vi "Main.vi"() -> ()   [LabVIEW 2013]
uses:
  <vilib>/Platform/TimedLoop/XDataNode/timing_clust.ctl
  <vilib>/Platform/TimedLoop/XDataNode/nitl_modes.ctl
  <vilib>/Platform/TimedLoop/XDataNode/wakeup.ctl
  <vilib>/DAQmx/read.llb/DAQmx Read (Analog 1D Wfm NChan NSamp).vi
  <vilib>/Analysis/2dsp.llb/Real FFT.vi
  <vilib>/DAQmx/create/channels.llb/DAQmx Create Channel (AI-Voltage-Basic).vi
  <vilib>/DAQmx/configure/timing.llb/DAQmx Timing (Sample Clock).vi
  <vilib>/addons/database/Connection.llb/DB Tools Open Connec (Path).vi
  <vilib>/Waveform/WDTOps.llb/WDT Index Channel DBL.vi
  <vilib>/measure/mamon.llb/Trigger Detection for 1 Channel.vi
  <vilib>/Waveform/WDTOps.llb/WDT Get Waveform Subset DBL.vi
  <vilib>/DAQmx/miscellaneous.llb/DAQmx Fill In Error Info.vi
  <vilib>/platform/TimedLoop/XDataNode/XDataNode.xnode
  <vilib>/addons/database/_DB Variant To Data/Database Variant To Data.xnode
  <vilib>/measure/NI_MAPro.lvlib
  <resource>/objmgr/daqmx.rc
  <vilib>/Analysis/NI_AALPro.lvlib
  <vilib>/addons/database/NI_Database_API.lvlib
  <vilib>/Platform/TimedLoop/XDataNode/XDNodeRunTimeDep.lvlib
panel:
  out "FFT 2":cluster{"t":dbl, dbl, dbl[]}(graph)
  in  "Canal 2":enum32{"DB"}(tab)
  in  "DB Retrieve 2":bool
  in  "Tabla 3":u16(ring) items=["Mediciones", "Pruebas"]
  in  "Título 4":u16(ring) items=["-", "fallo1", "fallo2", "fallo3"]
  in  "Remove":bool
  in  "Refresh":bool caption="Refresh Button"
  in  "Canal 1":enum32{"Page 1"}(tab)
  in  "DB Guardar":enum32{"DB"}(tab)
  in  "Tabla":u16(ring) items=["Mediciones", "Pruebas"]
  in  "Guardar":bool
  in  "Título":string="Saw"
  in  "Daq o DB":enum32{"DAQ", "DB"}(tab)
  in  "1 o Continuo":enum32{"Radio Selection 1", "Radio Selection 2"}(radio)
  in  "Play":bool
  in  "En Tiempo":bool
  in  "Tabla":u16(ring) items=["Mediciones", "Pruebas"]
  in  "Título":u16(ring) items=["-", "fallo1", "fallo2", "fallo3"]
  in  "DB Retrieve":bool
  out "F o T":enum32{"Frecuencia", "Tiempo"}(tab)
  out "FFT":cluster{"t":dbl, dbl, dbl[]}[](graph)
  out "Waveforms":waveform(dbl)[](graph)
  out "Waveform CMP":waveform(dbl)(graph)
  out "Waveform Inyector":waveform(dbl)(graph)
  out "Waveform Acelerometer":waveform(dbl)(graph)
  in  "stop":bool
  out "RPM":dbl
  out "error out":errorcluster
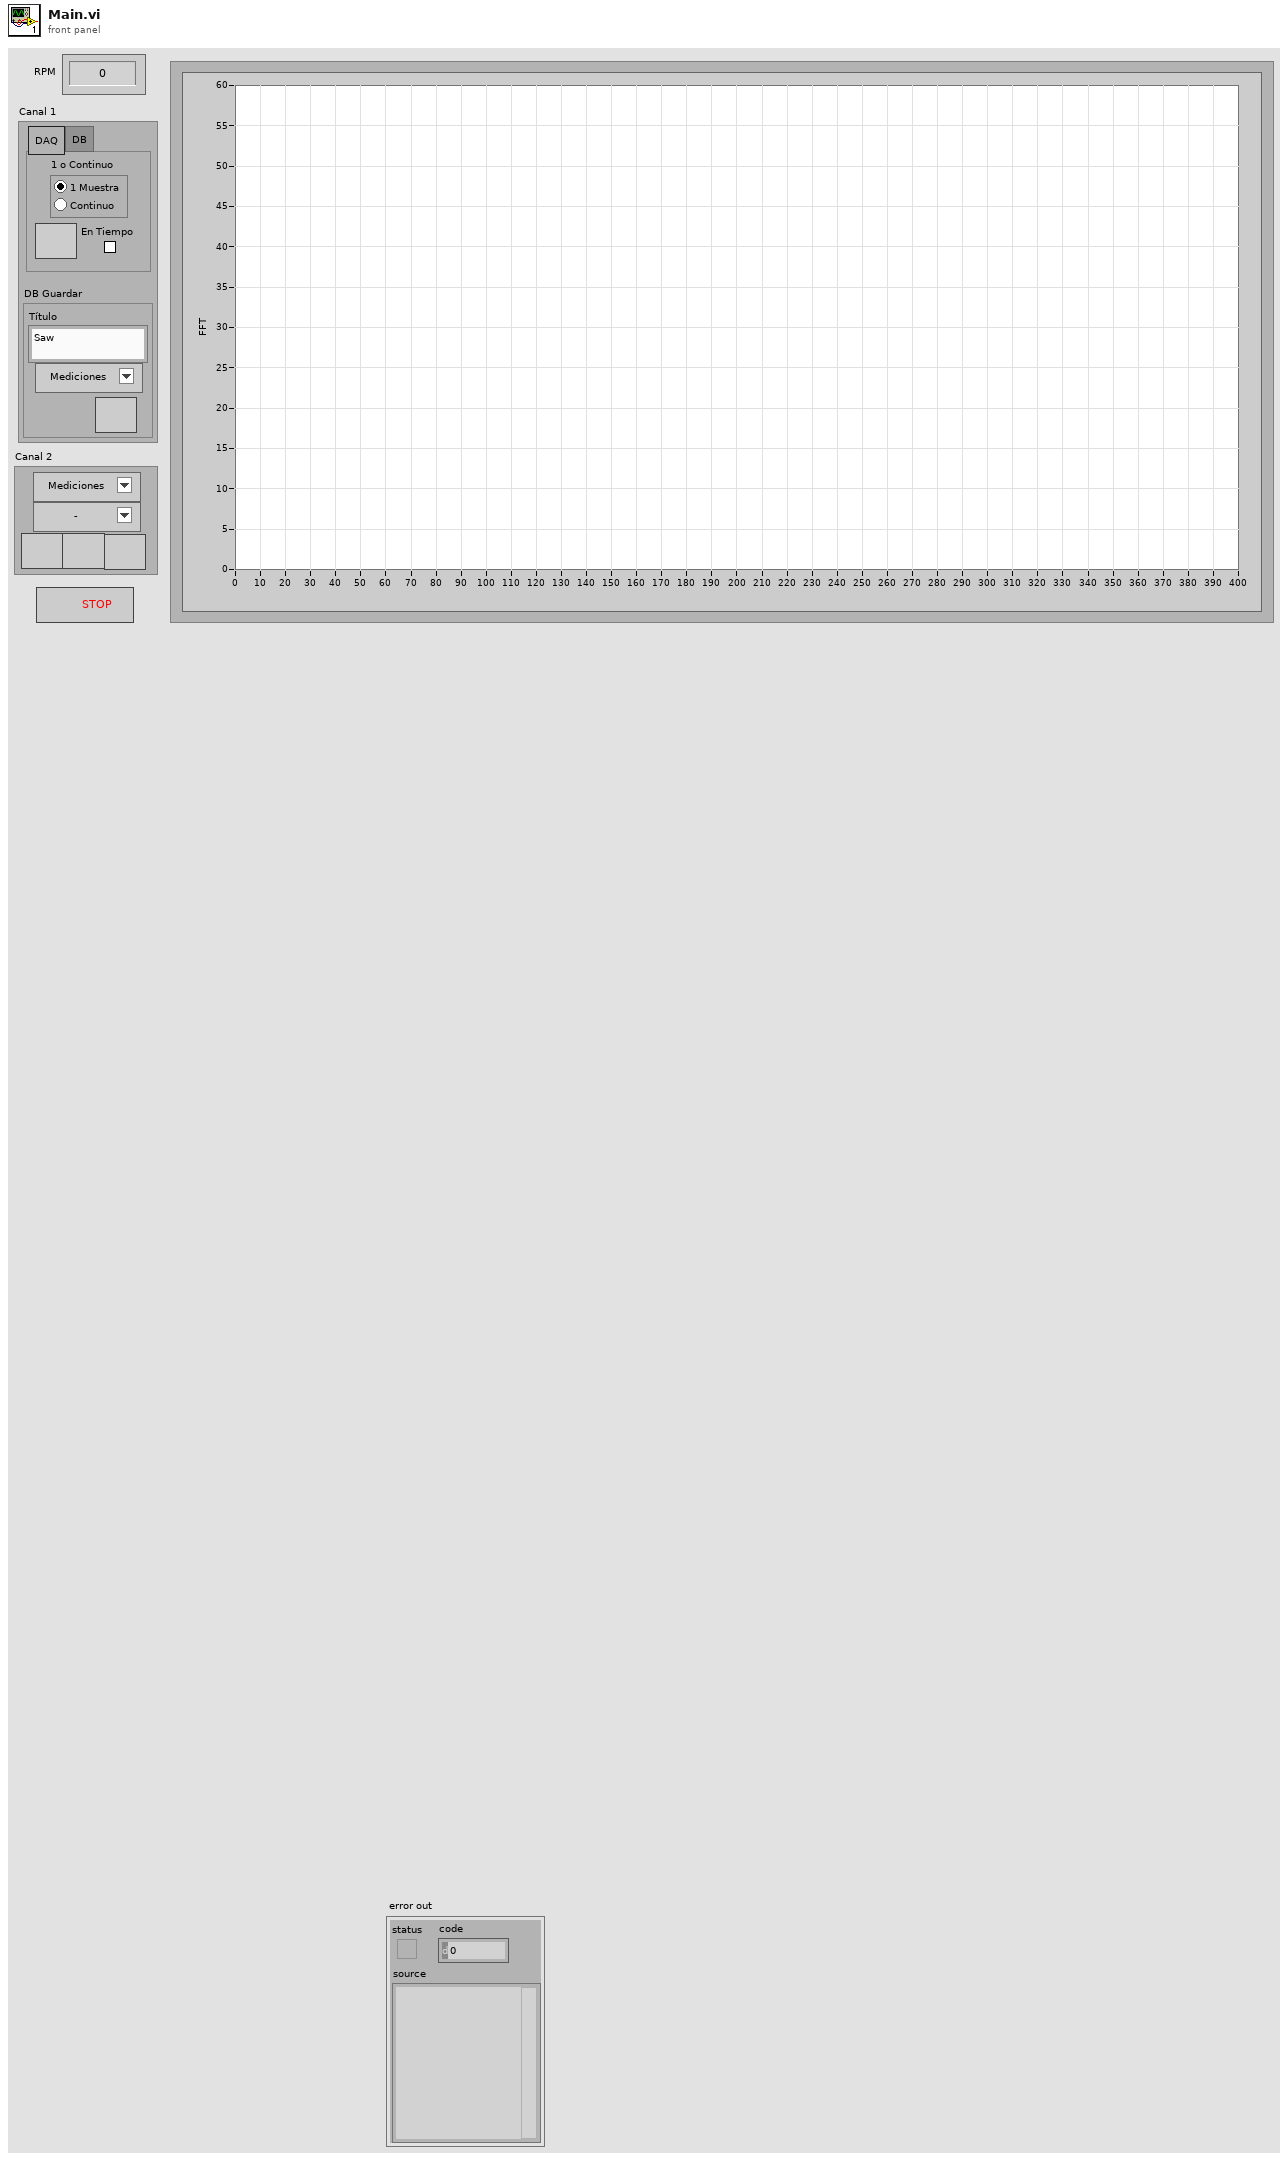
[diagram p1: front panel]
types:
  T1 = typedef "NI_Database_API.lvlib/Conn ObjectReference.ctl" = refnum<k1>
  T2 = cluster{"Título":string, cluster{"t":dbl, dbl, dbl[]}}
  T3 = typedef "XDNodeRunTimeDep.lvlib/timing_clust.ctl" = cluster{"Expected End [f-1]":u64, "Actual End [f-1]":u64, "Finished Late? [f-1]":bool, "Expected End [i-1]":u64, "Actual End [i-1]":u64, "Finished Late? [i-1]":bool, "Expected Start [i]":u64, "Actual Start [i]":u64, "Expected Start [f]":u64, "Actual Start [f]":u64, "Source Name":string, "Structure Name":string, "Period":i64, "Deadline":i64, "Offset":i64, "Start":i64, "Priority":i32, "Timeout":i32, "Mode":T4, "Wakeup Reason":T5, "Error":errorcluster, "Source Type":string, "Secondary Source Type":string, "Global End Time":u64, "Global Start Time":u64, "Frame Duration":u64, "Iteration Duration":u64, "Assigned CPU":i32, "I/O Scan Engine Mode":u32}
  T4 = typedef "XDNodeRunTimeDep.lvlib/nitl_modes.ctl" = enum32{"No Change", "Process missed periods, maintain original phase", "Discard missed periods, maintain original phase", "Process missed periods, ignore original phase", "Discard missed periods, ignore original phase"}
  T5 = typedef "XDNodeRunTimeDep.lvlib/wakeup.ctl" = enum32{"Normal", "Aborted", "Asynchronous wakeup", "Timing source error", "Timed loop error", "Timeout"}
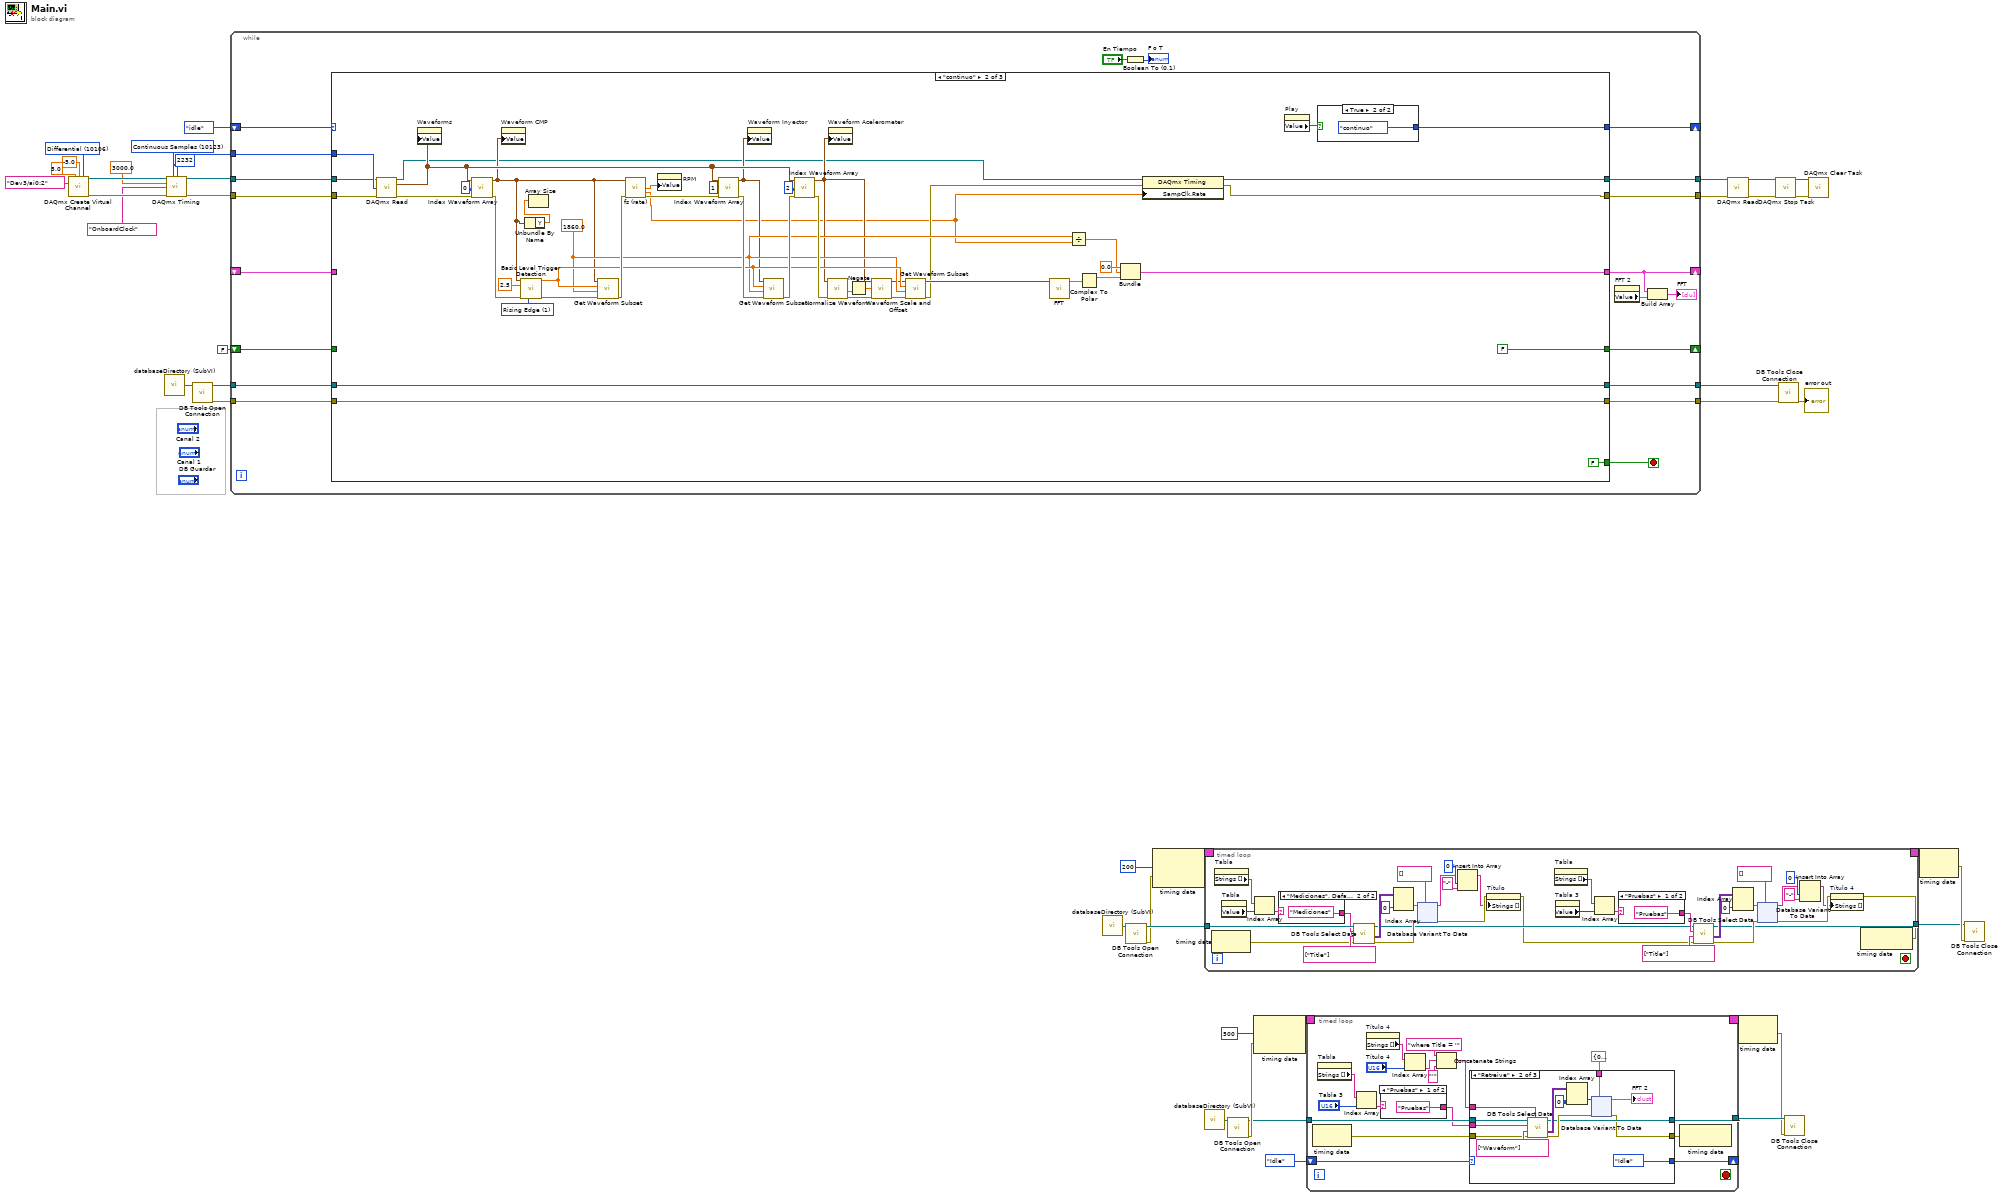
[diagram p0: block diagram]
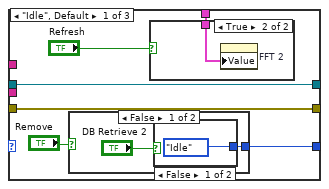
[diagram p2: hidden frame]
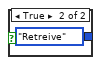
[diagram p4: hidden frame]
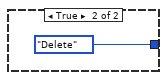
[diagram p5: hidden frame]
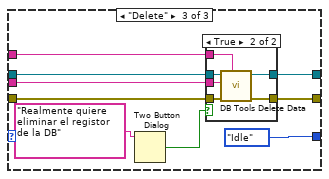
[diagram p6: hidden frame]
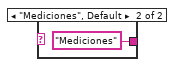
[diagram p8: hidden frame]
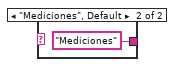
[diagram p9: hidden frame]
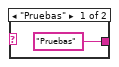
[diagram p10: hidden frame]
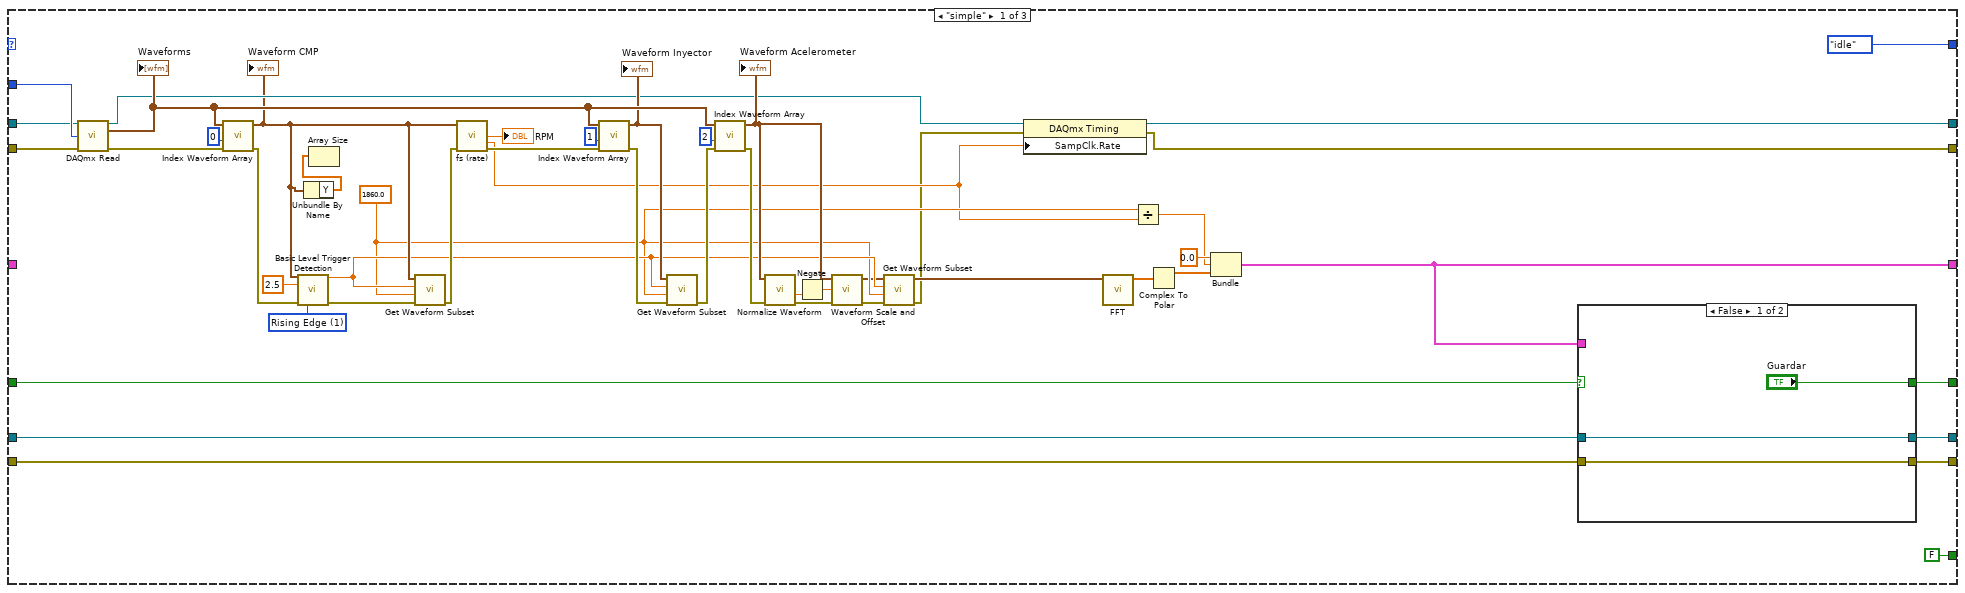
[diagram p11: hidden frame]
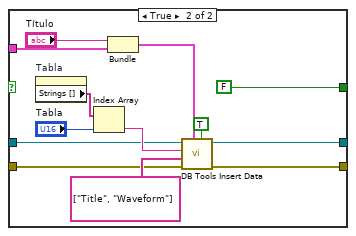
[diagram p12: hidden frame]
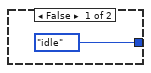
[diagram p13: hidden frame]
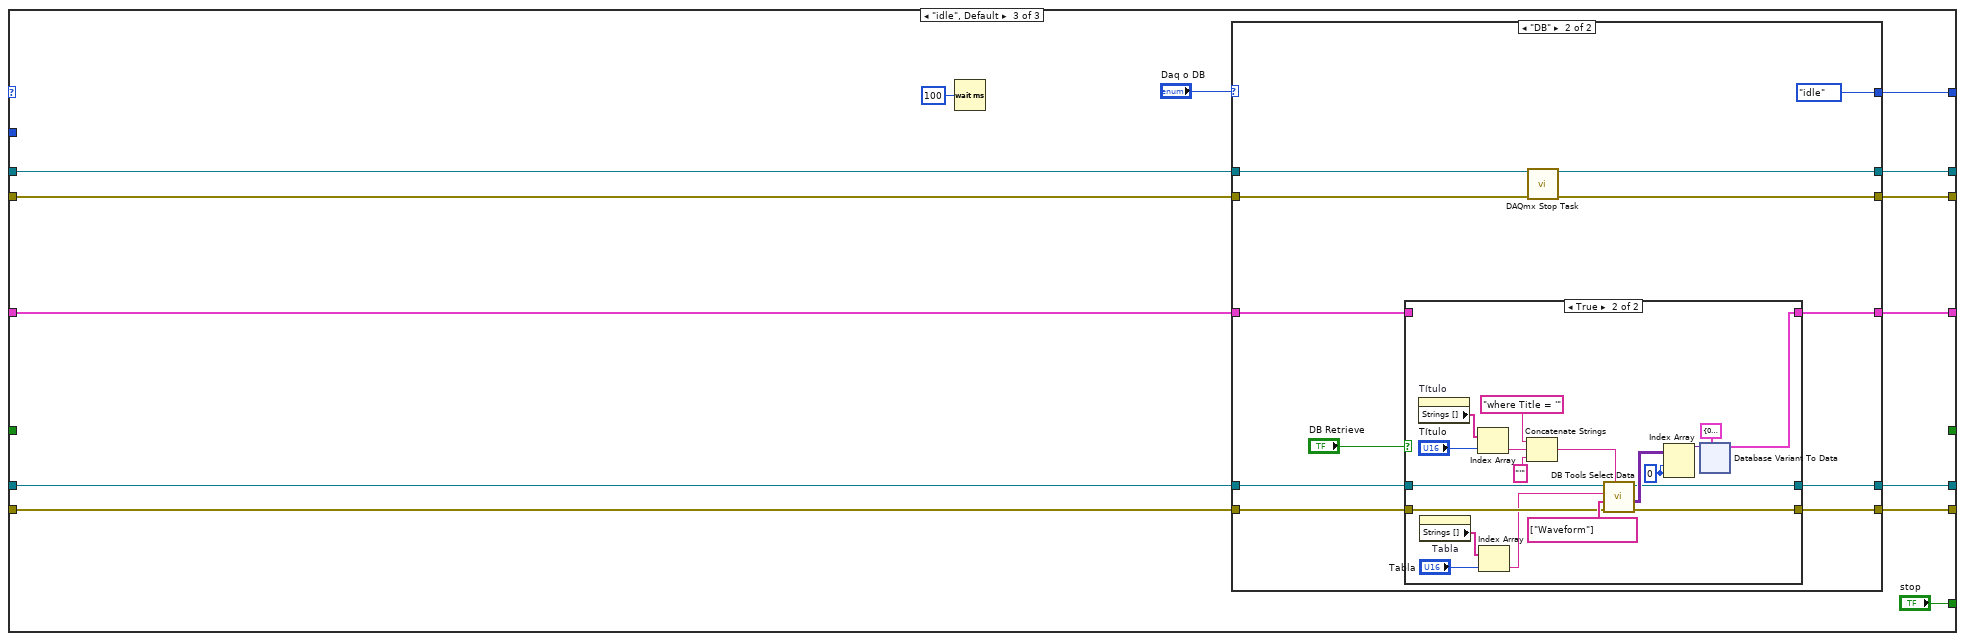
[diagram p14: hidden frame]
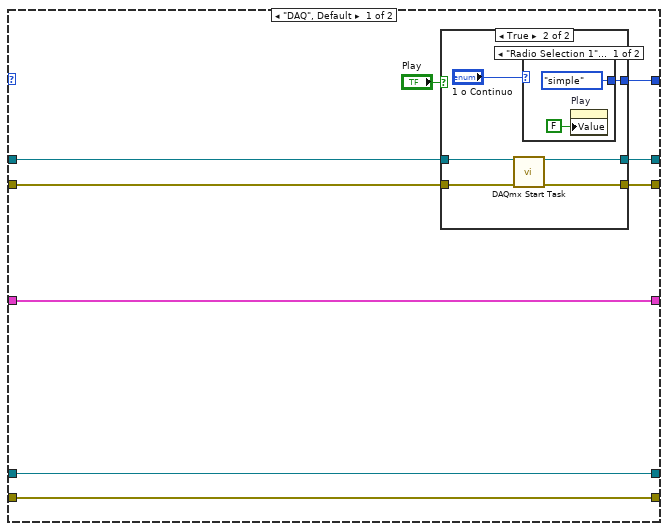
[diagram p15: hidden frame]
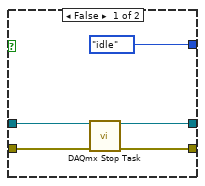
[diagram p16: hidden frame]
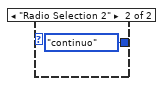
[diagram p17: hidden frame]
diagram:
  w37 = 10123 items=["Finite Samples"=10178, "Continuous Samples"=10123, "Hardware Timed Single Point"=12522] ("sample mode")
  w35 = 2232 ("samples per channel")
  w40 = 10106 items=["default"=-1, "RSE"=10083, "NRSE"=10078, "Differential"=10106, "Pseudodifferential"=12529] ("input terminal configuration")
  n1 = call-poly <vilib>:"DAQmx Create Virtual Channel.vi"("maximum value"=5.0, "minimum value"=-5.0, "input terminal configuration"=w40, "physical channels"=tag "Dev3/ai0:2") -> ("task out"=w39:refnum<k21>, "error out"=w38:errorcluster)  [unwired: 5 in, 5 out]
  n2 = call "databaseDirectory (SubVI).vi"() -> ("Application Directory"=w30:path)  [unwired: 1 in]
  n3 = call-poly <vilib>:"DAQmx Timing.vi"("task/channels in"=w39, "sample mode"=w37, "samples per channel"=w35, "rate"=3000.0, "source"=tag "OnboardClock", "error in"=w38) -> ("task out"=w23:refnum<k21>, "error out"=w22:errorcluster)  [unwired: 1 in, 7 out]
  n4 = call-poly <vilib>:"DB Tools Open Connection.vi"("connection information"=w30) -> ("error out"=w28:errorcluster, "connection reference"=w29:T1)  [unwired: 7 in]
  n5 = while {
    tunnel: w22 -> [w62]
    tunnel: w23 -> [w61]
    tunnel: [w60] -> w4
    tunnel: [w59] -> w2
    tunnel: w35 -> [w63]
    shift-right: [w58] -> _
    shift-left: FALSE ("OK Button") -> [w57]
    tunnel: w29 -> [w56]
    tunnel: w28 -> [w55]
    tunnel: [w54] -> w26
    tunnel: [w53] -> w25
    shift-right: [w51] -> _
    shift-left: enum32{"idle", "simple", "continuo"}."idle" ("Daq o DB") -> [w52]
    shift-right: [w48] -> _
    shift-left: _ -> [w45]
    stop <- w44 stop-if-true
    n6 = case shown="\"continuo\"" w52 {
      tunnel: w63 -> [w107 w169 _]
      tunnel: w62 -> [w89 w155 w180]
      tunnel: w61 -> [w88 w154 w181]
      tunnel: [w86 w130 w181] -> w60
      tunnel: [w85 w129 w180] -> w59
      tunnel: [w72 FALSE ("OK Button") _] -> w58
      tunnel: w57 -> [w71 _ _]
      tunnel: w56 -> [w70 w141 w185]
      tunnel: w55 -> [w69 w140 w182]
      tunnel: [w68 w141 w184] -> w54
      tunnel: [w67 w140 w183] -> w53
      tunnel: [enum32{"idle", "simple", "continuo"}."idle" ("Daq o DB") w143 w186] -> w51
      tunnel: [w65 w134 w177] -> w48
      tunnel: w45 -> [_ _ w178]
      tunnel: [FALSE ("stop") FALSE ("stop") "stop"] -> w44
      frame "simple" {
        w81 = 1860.0 ("duration")
        w110 = u16 1 items=["Falling Edge", "Rising Edge"] ("trigger slope")
        n7 = call-poly <vilib>:"DAQmx Read.vi"("task/channels in"=w88, "number of samples per channel"=w107, "error in"=w89) -> ("task out"=w87:refnum<k21>, "data"=w100:waveform(dbl)[], "error out"=w102:errorcluster)  [unwired: 10 out]
        "Waveforms" <- w100
        n8 = call-poly <vilib>:"Index Waveform Array.vi"("error in (no error)"=w102, "index"=0, "waveform array"=w100) -> ("error out"=w99:errorcluster, "waveform"=w84:waveform(dbl))  [unwired: 7 in]
        "Waveform CMP" <- w84
        n9 = call-poly <vilib>:"Basic Level Trigger Detection.vi"("signal in"=w84, "level"=2.5, "error in (no error)"=w99, "trigger slope"=w110) -> ("trigger location"=w82:dbl, "error out"=w98:errorcluster)  [unwired: 9 in, 1 out]
        n10 = Unbundle By Name(w84) -> ("Y"=w83:dbl[])
        n11 = Array Size(array=w83) -> ()  [unwired: 1 out]
        n12 = call-poly <vilib>:"Get Waveform Subset.vi"("error in (no error)"=w98, "duration"=w81, "start samples/time"=w82, "waveform in"=w84) -> ("error out"=w97:errorcluster)  [unwired: 2 in, 3 out]
        n13 = call "fs (rate).vi"("Waveform"=w84, "error in (no error)"=w97) -> ("rpm"=→"RPM":dbl, "fs (rate)"=w80:dbl, "error out"=w103:errorcluster)  [unwired: 9 in, 2 out]
        n14 = call-poly <vilib>:"Index Waveform Array.vi"("error in (no error)"=w103, "index"=1, "waveform array"=w100) -> ("error out"=w96:errorcluster, "waveform"=w94:waveform(dbl))  [unwired: 7 in]
        "Waveform Inyector" <- w94
        n15 = call-poly <vilib>:"Get Waveform Subset.vi"("error in (no error)"=w96, "duration"=w81, "start samples/time"=w82, "waveform in"=w94) -> ("error out"=w95:errorcluster)  [unwired: 2 in, 3 out]
        n16 = call-poly <vilib>:"Index Waveform Array.vi"("error in (no error)"=w95, "index"=2, "waveform array"=w100) -> ("error out"=w91:errorcluster, "waveform"=w90:waveform(dbl))  [unwired: 7 in]
        "Waveform Acelerometer" <- w90
        n17 = call <vilib>:"Normalize Waveform.vi"("error in (no error)"=w91, "waveform in"=w90) -> ("error out"=w93:errorcluster, "offset"=w79:dbl)  [unwired: 6 in, 2 out]
        n18 = Negate(x=w79) -> (-x=w78:dbl)
        n19 = call <vilib>:"Waveform Scale and Offset.vi"("error in (no error)"=w93, "offset"=w78, "waveform in"=w90) -> ("error out"=w92:errorcluster, "waveform out"=w77:waveform(dbl))  [unwired: 7 in]
        n20 = call-poly <vilib>:"Get Waveform Subset.vi"("error in (no error)"=w92, "duration"=w81, "start samples/time"=w82, "waveform in"=w77) -> ("error out"=w73:errorcluster, "waveform out"=w75:waveform(dbl))  [unwired: 2 in, 2 out]
        n21 = property class="DAQmx Timing"(reference=w87, error in=w73, "SampClk.Rate"=w80) -> (reference out=w86:refnum<k21>, error out=w85:errorcluster)
        n22 = call-poly <vilib>:"FFT.vi"("X"=w75) -> ("FFT {X}"=w76:cdb[])  [unwired: 9 in, 1 out]
        n23 = Divide(x=w81, y=w80) -> (x/y=w108:dbl)
        n24 = Complex To Polar(r * e^(i*theta)=w76) -> (r=w74:dbl[])  [unwired: 1 out]
        n25 = Bundle("t"=0.0, w108, w74) -> (w65:cluster{"t":dbl, dbl, dbl[]})  [unwired: 1 in]
        n26 = case shown="False" w71 {
          tunnel: ["Guardar" FALSE ("OK Button")] -> w72
          tunnel: w65 -> [_ w119]
          tunnel: w70 -> [w113 w118]
          tunnel: w69 -> [w112 w117]
          tunnel: [w113 w116] -> w68
          tunnel: [w112 w115] -> w67
          frame False {
          }
          frame True {
            n27 = property on="Tabla" class="Ring (strict)"() -> ("Strings []"=w122:string[])  [unwired: 2 in, 2 out]
            n28 = Index Array(array=w122, index="Tabla") -> (element=w120:string)
            n29 = Bundle("Título"="Título", w119) -> (w124:T2)  [unwired: 1 in]
            n30 = call <vilib>:"DB Tools Insert Data.vi"("create table? (F)"=TRUE ("create table? (f)"), "data"=w124, "error in (no error)"=w117, "columns"=string[] ["Title", "Waveform"], "table"=w120, "connection reference"=w118) -> ("error out"=w115:errorcluster, "connection reference out"=w116:T1)  [unwired: 4 in]
          }
        }
      }
      frame "continuo" {
        w151 = 1860.0 ("duration")
        w172 = u16 1 items=["Falling Edge", "Rising Edge"] ("trigger slope")
        n31 = call-poly <vilib>:"DAQmx Read.vi"("task/channels in"=w154, "number of samples per channel"=w169, "error in"=w155) -> ("task out"=w133:refnum<k21>, "data"=w138:waveform(dbl)[], "error out"=w165:errorcluster)  [unwired: 10 out]
        n32 = property on="Waveforms" class="WFGraph (strict)"("Value"=w138) -> ()  [unwired: 2 in, 2 out]
        n33 = call-poly <vilib>:"Index Waveform Array.vi"("error in (no error)"=w165, "index"=0, "waveform array"=w138) -> ("error out"=w163:errorcluster, "waveform"=w137:waveform(dbl))  [unwired: 7 in]
        n34 = property on="Waveform CMP" class="WFGraph (strict)"("Value"=w137) -> ()  [unwired: 2 in, 2 out]
        n35 = call-poly <vilib>:"Basic Level Trigger Detection.vi"("signal in"=w137, "level"=2.5, "error in (no error)"=w163, "trigger slope"=w172) -> ("trigger location"=w152:dbl, "error out"=w162:errorcluster)  [unwired: 9 in, 1 out]
        n36 = Unbundle By Name(w137) -> ("Y"=w153:dbl[])
        n37 = Array Size(array=w153) -> ()  [unwired: 1 out]
        n38 = call-poly <vilib>:"Get Waveform Subset.vi"("error in (no error)"=w162, "duration"=w151, "start samples/time"=w152, "waveform in"=w137) -> ("error out"=w161:errorcluster)  [unwired: 2 in, 3 out]
        n39 = call "fs (rate).vi"("Waveform"=w137, "error in (no error)"=w161) -> ("rpm"=w139:dbl, "fs (rate)"=w131:dbl, "error out"=w166:errorcluster)  [unwired: 9 in, 2 out]
        n40 = property on="RPM" class="DigNum (strict)"("Value"=w139) -> ()  [unwired: 2 in, 2 out]
        n41 = call-poly <vilib>:"Index Waveform Array.vi"("error in (no error)"=w166, "index"=1, "waveform array"=w138) -> ("error out"=w160:errorcluster, "waveform"=w136:waveform(dbl))  [unwired: 7 in]
        n42 = property on="Waveform Inyector" class="WFGraph (strict)"("Value"=w136) -> ()  [unwired: 2 in, 2 out]
        n43 = call-poly <vilib>:"Get Waveform Subset.vi"("error in (no error)"=w160, "duration"=w151, "start samples/time"=w152, "waveform in"=w136) -> ("error out"=w159:errorcluster)  [unwired: 2 in, 3 out]
        n44 = call-poly <vilib>:"Index Waveform Array.vi"("error in (no error)"=w159, "index"=2, "waveform array"=w138) -> ("error out"=w156:errorcluster, "waveform"=w135:waveform(dbl))  [unwired: 7 in]
        n45 = call <vilib>:"Normalize Waveform.vi"("error in (no error)"=w156, "waveform in"=w135) -> ("error out"=w158:errorcluster, "offset"=w150:dbl)  [unwired: 6 in, 2 out]
        n46 = property on="Waveform Acelerometer" class="WFGraph (strict)"("Value"=w135) -> ()  [unwired: 2 in, 2 out]
        n47 = Negate(x=w150) -> (-x=w149:dbl)
        n48 = call <vilib>:"Waveform Scale and Offset.vi"("error in (no error)"=w158, "offset"=w149, "waveform in"=w135) -> ("error out"=w157:errorcluster, "waveform out"=w148:waveform(dbl))  [unwired: 7 in]
        n49 = call-poly <vilib>:"Get Waveform Subset.vi"("error in (no error)"=w157, "duration"=w151, "start samples/time"=w152, "waveform in"=w148) -> ("error out"=w132:errorcluster, "waveform out"=w146:waveform(dbl))  [unwired: 2 in, 2 out]
        n50 = call-poly <vilib>:"FFT.vi"("X"=w146) -> ("FFT {X}"=w147:cdb[])  [unwired: 9 in, 1 out]
        n51 = Divide(x=w151, y=w131) -> (x/y=w170:dbl)
        n52 = Complex To Polar(r * e^(i*theta)=w147) -> (r=w145:dbl[])  [unwired: 1 out]
        n53 = Bundle("t"=0.0, w170, w145) -> (w134:cluster{"t":dbl, dbl, dbl[]})  [unwired: 1 in]
        n54 = property class="DAQmx Timing"(reference=w133, error in=w132, "SampClk.Rate"=w131) -> (reference out=w130:refnum<k21>, error out=w129:errorcluster)
        n55 = property on="Play" class="Bool (strict)"() -> ("Value"=w142:bool)  [unwired: 2 in, 2 out]
        n56 = case shown="True" w142 {
          tunnel: [enum32{"idle", "simple", "continuo"}."idle" ("Daq o DB") enum32{"idle", "simple", "continuo"}."continuo" ("Daq o DB")] -> w143
          frame False {
          }
          frame True {
          }
        }
      }
      frame "idle", Default {
        n57 = Wait (ms)(milliseconds to wait=u32 100) -> ()  [unwired: 1 out]
        n58 = case shown="\"DB\"" "Daq o DB" {
          tunnel: [w195 enum32{"idle", "simple", "continuo"}."idle" ("Daq o DB")] -> w186
          tunnel: w185 -> [w194 w220]
          tunnel: [w194 w218] -> w184
          tunnel: [w193 w217] -> w183
          tunnel: w182 -> [w193 w219]
          tunnel: w181 -> [w192 w216]
          tunnel: [w191 w215] -> _
          tunnel: w180 -> [w190 w214]
          tunnel: [w189 w213] -> _
          tunnel: w178 -> [w188 w212]
          tunnel: [w188 w211] -> w177
          frame "DAQ", Default {
            n59 = case shown="True" "Play" {
              tunnel: [enum32{"idle", "simple", "continuo"}."idle" ("Daq o DB") w207] -> w195
              tunnel: w192 -> [w200 w204]
              tunnel: [w197 w203] -> w191
              tunnel: w190 -> [w199 w205]
              tunnel: [w198 w202] -> w189
              frame False {
                n60 = call <vilib>:"DAQmx Stop Task.vi"("task/channels in"=w200, "error in"=w199) -> ("task out"=w197:refnum<k21>, "error out"=w198:errorcluster)  [unwired: 12 out]
              }
              frame True {
                n61 = call <vilib>:"DAQmx Start Task.vi"("task/channels in"=w204, "error in"=w205) -> ("task out"=w203:refnum<k21>, "error out"=w202:errorcluster)  [unwired: 12 out]
                n62 = case shown="\"Radio Selection 1\", Default" "1 o Continuo" {
                  tunnel: [enum32{"idle", "simple", "continuo"}."simple" ("Daq o DB") enum32{"idle", "simple", "continuo"}."continuo" ("Daq o DB")] -> w207
                  frame "Radio Selection 1", Default {
                    n63 = property on="Play" class="Bool (strict)"("Value"=FALSE ("Play")) -> ()  [unwired: 2 in, 2 out]
                  }
                  frame "Radio Selection 2" {
                  }
                }
              }
            }
          }
          frame "DB" {
            n64 = case shown="True" "DB Retrieve" {
              tunnel: w220 -> [w225 w232]
              tunnel: [w225 w230] -> w218
              tunnel: w219 -> [w224 w231]
              tunnel: [w224 w229] -> w217
              tunnel: w212 -> [w223 _]
              tunnel: [w223 w228] -> w211
              frame False {
              }
              frame True {
                w233 = 0 ("index")
                n65 = property on="Título" class="Ring (strict)"() -> ("Strings []"=w243:string[])  [unwired: 2 in, 2 out]
                n66 = property on="Tabla" class="Ring (strict)"() -> ("Strings []"=w241:string[])  [unwired: 2 in, 2 out]
                n67 = Index Array(array=w243, index="Título") -> (element=w227:string)
                n68 = Index Array(array=w241, index="Tabla") -> (element=w226:string)
                n69 = Concatenate Strings("where Title = '" ("condition"), w227, "'" ("condition")) -> (w240:string)
                n70 = call <vilib>:"DB Tools Select Data.vi"("condition"=w240, "error in (no error)"=w231, "columns"=string[] ["Waveform"], "table"=w226, "connection reference"=w232) -> ("error out"=w229:errorcluster, "data"=w234:variant[][], "connection reference out"=w230:T1)  [unwired: 1 in]
                n71 = Index Array(array=w234, index (row)=w233, index (col)=w233) -> (element=w235:variant)
                n72 = xnode "Database Variant To Data"("database variant"=w235, "type"=cluster{"t":dbl, dbl, dbl[]} {"t"=0.0, 0.0, []}) -> ("data"=w228:cluster{"t":dbl, dbl, dbl[]})  [unwired: 1 in, 1 out]
              }
            }
            n73 = call <vilib>:"DAQmx Stop Task.vi"("task/channels in"=w216, "error in"=w214) -> ("task out"=w215:refnum<k21>, "error out"=w213:errorcluster)  [unwired: 12 out]
          }
        }
      }
    }
    n74 = Boolean To (0,1)(Boolean="En Tiempo") -> (0, 1=→"F o T":i16)
    n75 = property on="FFT 2" class="WFGraph (strict)"() -> ("Value"=w46:cluster{"t":dbl, dbl, dbl[]})  [unwired: 2 in, 2 out]
    n76 = Build Array(w48, w46) -> (→"FFT":cluster{"t":dbl, dbl, dbl[]}[])
  }
  n77 = call "databaseDirectory (SubVI).vi"() -> ("Application Directory"=w18:path)  [unwired: 1 in]
  n78 = call-poly <vilib>:"DB Tools Open Connection.vi"("connection information"=w18) -> ("error out"=w16:errorcluster, "connection reference"=w17:T1)  [unwired: 7 in]
  n79 = node-c288(i64 200 ("Period"), w16) -> (w21:T3)
  n80 = call "databaseDirectory (SubVI).vi"() -> ("Application Directory"=w8:path)  [unwired: 1 in]
  n81 = timed-loop {
    timing: w21 -> [_]
    timing-out: [_] -> w20
    tunnel: w17 -> [w315]
    tunnel: [w293] -> w14
    stop <- _ stop-if-true
    n82 = node-c288() -> (w304:errorcluster)  [unwired: 1 in]
    n83 = property on="Tabla" class="Ring (strict)"() -> ("Strings []"=w308:string[])  [unwired: 2 in, 2 out]
    n84 = property on="Tabla" class="Ring (strict)"() -> ("Value"=w307:u16)  [unwired: 2 in, 2 out]
    n85 = Index Array(array=w308, index=w307) -> (element=w306:string)
    n86 = case shown="\"Mediciones\", Default" w306 {
      tunnel: ["Pruebas" ("table") "Mediciones" ("table")] -> w305
      frame "Pruebas" {
      }
      frame "Mediciones", Default {
      }
    }
    n87 = call <vilib>:"DB Tools Select Data.vi"("error in (no error)"=w304, "columns"=string[] ["Title"], "table"=w305, "connection reference"=w315) -> ("error out"=w309:errorcluster, "data"=w312:variant[][], "connection reference out"=w295:T1)  [unwired: 2 in]
    n88 = Index Array(array=w312, index (col)=0 ("index")) -> (element=w311:variant[])  [unwired: 1 in]
    n89 = xnode "Database Variant To Data"("database variant"=w311, "error in (no error)"=w309, "type"=string[] []) -> ("data"=w285:string[], "error out"=w291:errorcluster)
    n90 = Insert Into Array(array=w285, index=0, new element="-" ("new element/subarray")) -> (w284:string[])
    n91 = property on="Título" class="Ring (strict)"(error in=w291, "Strings []"=w284) -> (error out=w290:errorcluster)  [unwired: 1 in, 1 out]
    n92 = property on="Tabla" class="Ring (strict)"() -> ("Strings []"=w301:string[])  [unwired: 2 in, 2 out]
    n93 = property on="Tabla 3" class="Ring (strict)"() -> ("Value"=w292:u16)  [unwired: 2 in, 2 out]
    n94 = Index Array(array=w301, index=w292) -> (element=w302:string)
    n95 = case shown="\"Pruebas\"" w302 {
      tunnel: ["Pruebas" ("table") "Mediciones" ("table")] -> w303
      frame "Pruebas" {
      }
      frame "Mediciones", Default {
      }
    }
    n96 = call <vilib>:"DB Tools Select Data.vi"("error in (no error)"=w290, "columns"=string[] ["Title"], "table"=w303, "connection reference"=w295) -> ("error out"=w294:errorcluster, "data"=w298:variant[][], "connection reference out"=w293:T1)  [unwired: 2 in]
    n97 = Index Array(array=w298, index (col)=0 ("index")) -> (element=w299:variant[])  [unwired: 1 in]
    n98 = xnode "Database Variant To Data"("database variant"=w299, "error in (no error)"=w294, "type"=string[] []) -> ("data"=w281:string[], "error out"=w289:errorcluster)
    n99 = Insert Into Array(array=w281, index=0, new element="-" ("new element/subarray")) -> (w280:string[])
    n100 = property on="Título 4" class="Ring (strict)"(error in=w289, "Strings []"=w280) -> (error out=w288:errorcluster)  [unwired: 1 in, 1 out]
    n101 = node-c288(w288) -> ()  [unwired: 1 out]
  }
  n102 = call-poly <vilib>:"DB Tools Open Connection.vi"("connection information"=w8) -> ("error out"=w10:errorcluster, "connection reference"=w9:T1)  [unwired: 7 in]
  n103 = node-c288(i64 500 ("Period"), w10) -> (w13:T3)
  n104 = timed-loop {
    timing: w13 -> [_]
    timing-out: [_] -> w12
    tunnel: w9 -> [w417]
    tunnel: [w413] -> w11
    shift-right: [w403] -> _
    shift-left: enum16{"Idle", "Retreive", "Delete"}."Idle" -> [w404]
    stop <- _ stop-if-true
    n105 = node-c288() -> (w414:errorcluster)  [unwired: 1 in]
    n106 = property on="Tabla" class="Ring (strict)"() -> ("Strings []"=w412:string[])  [unwired: 2 in, 2 out]
    n107 = Index Array(array=w412, index="Tabla 3") -> (element=w416:string)
    n108 = property on="Título 4" class="Ring (strict)"() -> ("Strings []"=w410:string[])  [unwired: 2 in, 2 out]
    n109 = case shown="\"Pruebas\"" w416 {
      tunnel: ["Pruebas" ("table") "Mediciones" ("table")] -> w415
      frame "Pruebas" {
      }
      frame "Mediciones", Default {
      }
    }
    n110 = Index Array(array=w410, index="Título 4") -> (element=w411:string)
    n111 = Concatenate Strings("where Title = '" ("condition"), w411, "'" ("condition")) -> (w406:string)
    n112 = case shown="\"Retreive\"" w404 {
      tunnel: w417 -> [w423 w443 w485]
      tunnel: w415 -> [_ w438 w483]
      tunnel: w414 -> [w422 w437 w487]
      tunnel: [w423 w435 w484] -> w413
      tunnel: w406 -> [_ w434 w482]
      tunnel: [w422 w433 w486] -> w405
      tunnel: [w421 enum16{"Idle", "Retreive", "Delete"}."Idle" enum16{"Idle", "Retreive", "Delete"}."Idle"] -> w403
      tunnel: cluster{"t":dbl, dbl, dbl[]} {"t"=0.0, 0.0, []} -> [w418 w430 _]
      frame "Idle", Default {
        n113 = case shown="False" "Remove" {
          tunnel: [w426 enum16{"Idle", "Retreive", "Delete"}."Delete"] -> w421
          frame False {
            n114 = case shown="False" "DB Retrieve 2" {
              tunnel: [enum16{"Idle", "Retreive", "Delete"}."Idle" enum16{"Idle", "Retreive", "Delete"}."Retreive"] -> w426
              frame False {
              }
              frame True {
              }
            }
          }
          frame True {
          }
        }
        n115 = case shown="True" "Refresh" {
          tunnel: w418 -> [_ w424]
          frame False {
          }
          frame True {
            n116 = property on="FFT 2" class="WFGraph (strict)"("Value"=w424) -> ()  [unwired: 2 in, 2 out]
          }
        }
      }
      frame "Retreive" {
        w436 = 0 ("index")
        n117 = call <vilib>:"DB Tools Select Data.vi"("condition"=w434, "error in (no error)"=w437, "columns"=string[] ["Waveform"], "table"=w438, "connection reference"=w443) -> ("error out"=w439:errorcluster, "data"=w441:variant[][], "connection reference out"=w435:T1)  [unwired: 1 in]
        n118 = Index Array(array=w441, index (row)=w436, index (col)=w436) -> (element=w440:variant)
        n119 = xnode "Database Variant To Data"("database variant"=w440, "error in (no error)"=w439, "type"=w430) -> ("data"=→"FFT 2":cluster{"t":dbl, dbl, dbl[]}, "error out"=w433:errorcluster)
      }
      frame "Delete" {
        n120 = Two Button Dialog(message="Realmente quiere eliminar el registor de la DB") -> (T button?=w480:bool)  [unwired: 2 in]
        n121 = case shown="True" w480 {
          tunnel: w487 -> [w488 w495]
          tunnel: [w488 w494] -> w486
          tunnel: w485 -> [w489 w493]
          tunnel: [w489 w492] -> w484
          tunnel: w483 -> [_ w491]
          tunnel: w482 -> [_ w490]
          frame False {
          }
          frame True {
            n122 = call <vilib>:"DB Tools Delete Data.vi"("condition"=w490, "error in (no error)"=w495, "table"=w491, "connection reference"=w493) -> ("error out"=w494:errorcluster, "connection reference out"=w492:T1)  [unwired: 6 in]
          }
        }
      }
    }
    n123 = node-c288(w405) -> ()  [unwired: 1 out]
  }
  n124 = call-poly <vilib>:"DAQmx Read.vi"("task/channels in"=w4, "error in"=w2) -> ("task out"=w3:refnum<k21>, "error out"=w1:errorcluster)  [unwired: 1 in, 11 out]
  n125 = node-c288(w12) -> (w6:errorcluster)
  n126 = call <vilib>:"DAQmx Stop Task.vi"("task/channels in"=w3, "error in"=w1) -> ("task out"=w34:refnum<k21>, "error out"=w33:errorcluster)  [unwired: 12 out]
  n127 = call <vilib>:"DB Tools Close Connection.vi"("error in (no error)"=w25, "connection reference"=w26) -> ("error out"=→"error out":errorcluster)  [unwired: 5 in]
  n128 = call <vilib>:"DB Tools Close Connection.vi"("error in (no error)"=w6, "connection reference"=w11) -> ()  [unwired: 5 in, 1 out]
  n129 = call <vilib>:"DAQmx Clear Task.vi"("task in"=w34, "error in"=w33) -> ()  [unwired: 13 in, 1 out]
  n130 = node-c288(w20) -> (w15:errorcluster)
  n131 = call <vilib>:"DB Tools Close Connection.vi"("error in (no error)"=w15, "connection reference"=w14) -> ()  [unwired: 5 in, 1 out]
